vi "Array1.vi"() -> ()   [LabVIEW 2020]
panel:
  out "output array":dbl[](array[numeric])
  in  "new element/subarray":dbl
  out "element 3":dbl
  out "element 2":dbl
  in  "index 3":i32
  in  "index 2":i32
  out "element":dbl
  in  "index":i32
  out "size(s)":i32
  out "appended array":dbl[](array[numeric])
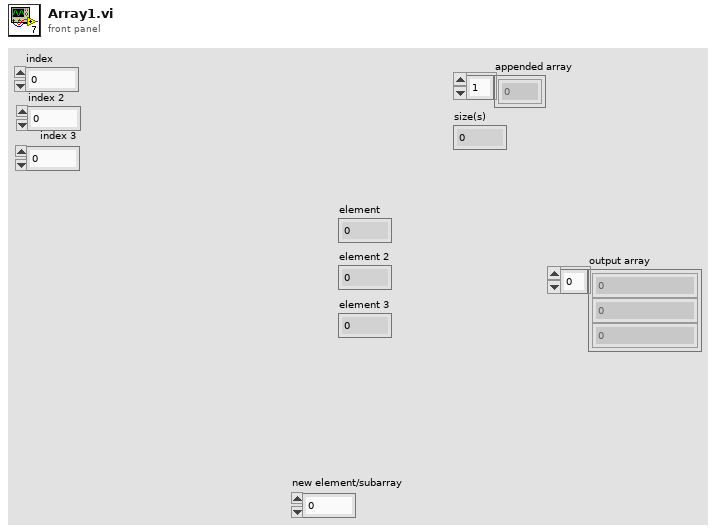
[diagram p1: front panel]
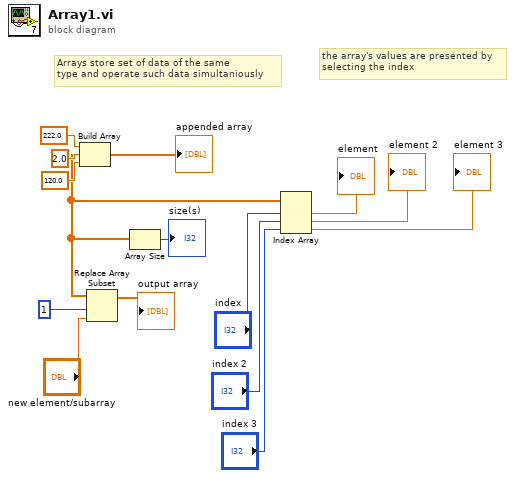
[diagram p0: block diagram]
diagram:
  # "the array's values are presented by \nselecting the index"
  # "Arrays store set of data of the same \ntype and operate such data simultaniously"
  n1 = Build Array(222.0 ("element"), 2.0 ("element"), 120.0 ("element")) -> (w4:dbl[])
  "appended array" <- w4
  n2 = Replace Array Subset(array=w4, new element="new element/subarray", index=1) -> (→"output array":dbl[])
  n3 = Array Size(array=w4) -> (size(s)=→"size(s)":i32)
  n4 = Index Array(array=w4, index #1="index", index #2="index 2", index #3="index 3") -> (element #1=→"element":dbl, element #2=→"element 2":dbl, element #3=→"element 3":dbl)
